vi "Ramp.vi"(9 "Slew Y":dbl=0.2, 10 "Output":bool, 11 "upper limit in":dbl) -> (3 "upper limit out":dbl)   [LabVIEW 2017]
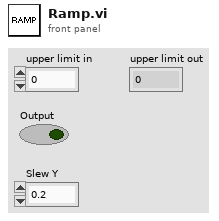
[diagram p1: front panel]
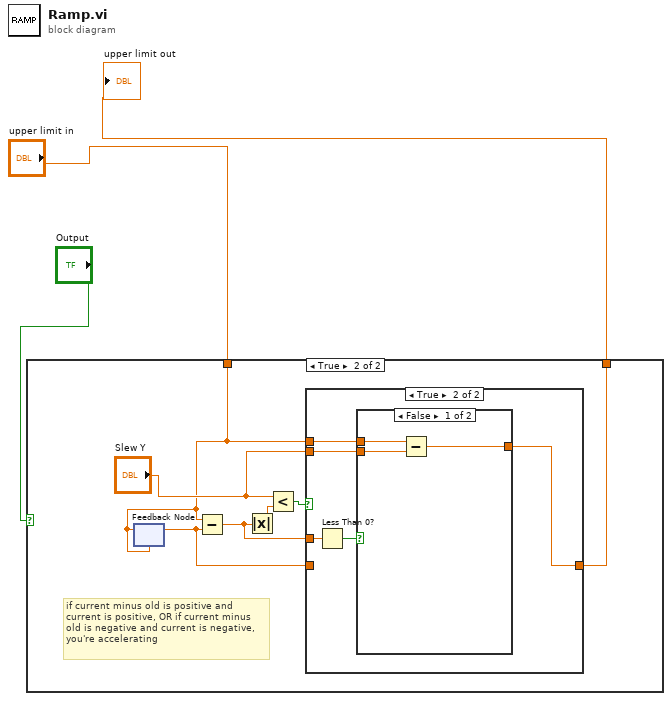
[diagram p0: block diagram]
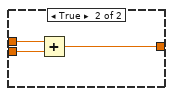
[diagram p4: hidden frame]
diagram:
  n1 = case shown="True" "Output" {
    tunnel: "upper limit in" -> [w4 w6]
    tunnel: [w4 w5] -> w2
    frame False {
    }
    frame True {
      # "if current minus old is positive and\ncurrent is positive, OR if current minus\nold is negative and current is negative,\nyou're accelerating"
      n2 = feedback #1(w6) -> (w8:dbl)
      n3 = feedback-in #1(w6) -> ()
      n4 = Subtract(x=w6, y=w8) -> (x-y=w9:dbl)
      n5 = Absolute Value(x=w9) -> (abs(x)=w11:dbl)
      n6 = Less?(x="Slew Y", y=w11) -> (x < y?=w10:bool)
      n7 = case shown="True" w10 {
        tunnel: [w12 w14] -> w5
        tunnel: w8 -> [w12 _]
        tunnel: w9 -> [_ w17]
        tunnel: w6 -> [_ w15]
        tunnel: "Slew Y" -> [_ w13]
        frame False {
        }
        frame True {
          n8 = Less Than 0?(x=w17) -> (x < 0?=w16:bool)
          n9 = case shown="False" w16 {
            tunnel: w15 -> [w20 w23]
            tunnel: [w19 w22] -> w14
            tunnel: w13 -> [w18 w21]
            frame False {
              n10 = Subtract(x=w20, y=w18) -> (x-y=w19:dbl)
            }
            frame True {
              n11 = Add(x=w23, y=w21) -> (x+y=w22:dbl)
            }
          }
        }
      }
    }
  }
  "upper limit out" <- w2
